vi "Ex1.vi"   [LabVIEW 2012]
panel:
  # "Hit run to nod the head"
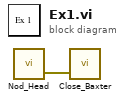
[diagram p0: block diagram]
diagram:
  n1 = call <userlib>:"Nod_Head.vi"() -> ("error out"=w1:errorcluster)  [unwired: 4 in]
  n2 = call <userlib>:"Close_Baxter.vi"("error in"=w1) -> ()  [unwired: 3 in, 1 out]
